vi "FastCMOSTestTrackerModule.vi"() -> ()   [LabVIEW 2011]
uses:
  qtrk/QTrk.llb/QTrkInstance.ctl
  qtrk/QTrk.llb/QTrkLocalizationResult.ctl
  qtrk/QTrk.llb/QTrkLocalizationJob.ctl
  qtrk/QTrk.llb/XYZf.ctl
  mkCameraData.ctl
  CameraConfig.ctl
  Main/Camera/GenericCameraConfigType.ctl
  qtrk/QTrk.llb/QTrkPixelDataType.ctl
  Main/GlobalVariables.vi
  qtrk/QTrk.llb/QTrkDLL.vi
panel:
  in  "Use frame-encoded\ntimestamp":bool
  out "Buffer numbers":i32[](graph)
  out "Buffer Number":i32
  in  "#frames to take":i32=50000
  out "Frame#":u32
  out "Z Result":sgl[](graph)
  out "Unsorted results":T1[](array[typedef])
  out "Results":T1[][](array[typedef])
  out "NumBeads":i32
  out "#frames":u32
  in  "Bead index":i32
  out "XY Result":sgl[][](graph)
  in  "Tracking enabled?":bool
  in  "stop":bool
  out "Status Information : Lost Frames":u32
  out "QTrk Instance":T4
  in  "Run grab sesh":bool
  in  "Stop":bool
  in  "Run":bool
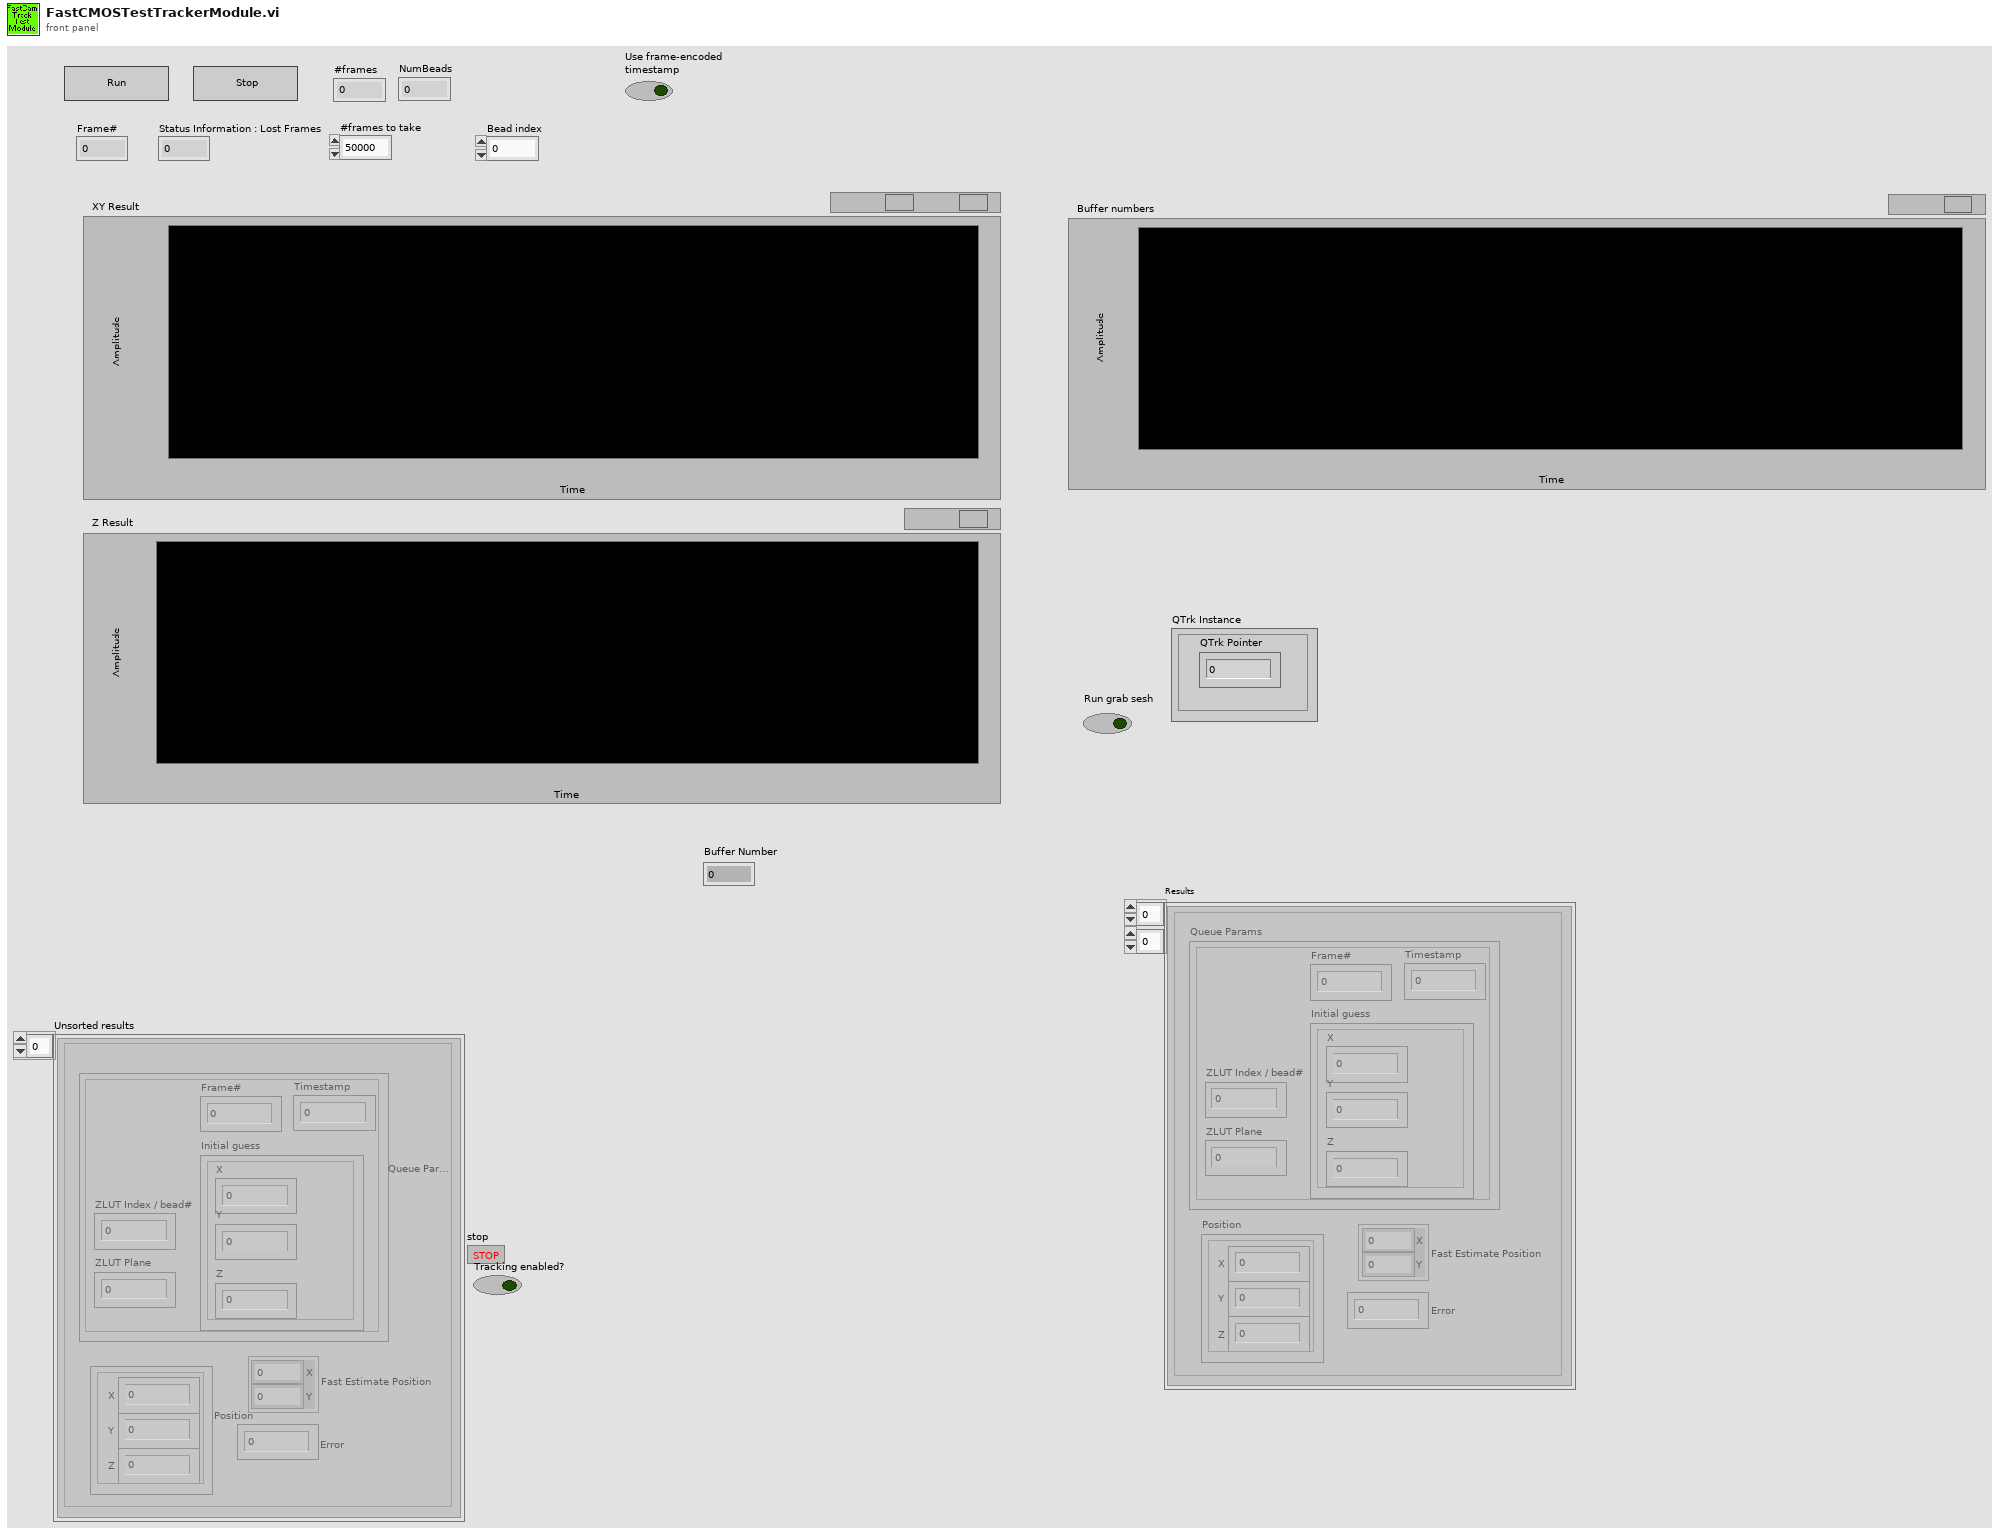
[diagram p1: front panel]
types:
  T1 = typedef "QTrkLocalizationResult.ctl" = cluster{"Queue Params":T2, "Position":T3, "Fast Estimate Position":cluster{"X":sgl, "Y":sgl}, "Error":i32}
  T2 = typedef "QTrkLocalizationJob.ctl" = cluster{"Frame#":u32, "Timestamp":u32, "ZLUT Index / bead#":i32, "ZLUT Plane":i32, "Initial guess":T3}
  T3 = typedef "XYZf.ctl" = cluster{"X":sgl, "Y":sgl, "Z":sgl}
  T4 = typedef "QTrkInstance.ctl" = cluster{"QTrk Pointer":u64}
  T5 = typedef "mkCameraData.ctl" = cluster{"Session":refnum<k11>, "Settings":T6}
  T6 = typedef "CameraConfig.ctl" = cluster{"Gain [1-4]":sgl, "Offset":i16, "Mode":i16, "ROIs":cluster{"X":i32, "Y":i32}[], "ROI Size":cluster{"X":i32, "Y":i32}, "Number of buffers":i32, "Use hardware multiple-ROI?":bool, "GenericCameraConfig":T7}
  T7 = typedef "GenericCameraConfigType.ctl" = cluster{"Framerate (Hz)":i32, "Exposure time (us)":i32, "Image size":cluster{"Width":i32, "Height":i32}, "Number of buffers":i32}
  T8 = enum16{"Use QTrk settings", "Select best device", "Use all devices", "Use custom list"}
  T9 = typedef "CameraInstance.ctl" = cluster{"VI refs":T10, "Camera state":variant}
  T10 = typedef "CameraInterface.ctl" = cluster{"Close":T11, "Get/Set generic config":T12, "Grab":T13, "Show Settings Dialog":T14, "AdjustBeadPos":T15, "Save/load camera settings":T16}
  T11 = typedef "CICloseType.ctl" = refnum<vi>
  T12 = typedef "CIGetSetGenericConfig.ctl" = refnum<vi>
  T13 = typedef "CIGrabType.ctl" = refnum<vi>
  T14 = typedef "CISettingsDlg.ctl" = refnum<vi>
  T15 = typedef "CIAdjustBeadPos.ctl" = refnum<vi>
  T16 = typedef "CISaveLoadSettings.ctl" = refnum<vi>
  T17 = typedef "MeasureConfigType.ctl" = cluster{"Bead locations":cluster{"X":i32, "Y":i32}[], "ROI":i32, "Experiment base path":path, "Image output subdir":string, "Output mode":T18, "Traces output subdir":string, "QTrk Settings":T19, "Tracking Config":T20, "Experiment Name":string, "Program":T23, "ZLUT":sgl[][][], "Camera settings":T7, "Experiment Script":string, "Max frames in memory":i32, "Save traces as binary":bool, "Pixel Calibration Gain Image":string, "Pixel Calibration Offset Image":string, "Use pixel calibration images":bool, "Internal camera settings":string}
  T18 = typedef "MeasureConfigOutputMode.ctl" = enum16{"None", "Track", "SaveImages"}
  T19 = typedef "QTrkSettings.ctl" = cluster{"Image width":i32, "Image height":i32, "Number of threads (CPU based)":i32, "CUDA Device":i32, "COM Background correction factor":sgl, "ZLUT MinRadius":sgl, "ZLUT Radial sample density":sgl, "ZLUT Angular sample density":sgl, "ZLUT ROI Coverage":sgl, "QI Iterations":i32, "QI MinRadius":sgl, "QI Radial sample density":sgl, "QI Angular sample density":sgl, "QI ROI Coverage":sgl, "QI Angular Step \nIteration Factor":sgl, "XCOR Profile Length":i32, "XCOR Profile Width":i32, "XCOR Iterations":i32, "Gaussian 2D Fit Iterations":i32, "Gaussian 2D Sigma (pixels)":sgl}
  T20 = typedef "TrackingConfigType.ctl" = cluster{"Number of steps":i32, "ZLUT stepsize (um)":sgl, "Z correction factor":sgl, "Start piezo Z (um)":sgl, "Pixel size (nm)":sgl, "2D Localization Type":T21, "Z Command (None)":T22, "Z Piezo scale":bool}
  T21 = typedef "QTrkLocalizationType.ctl" = enum16{"Center-of-Mass", "1D Cross-Correlation", "Quadrant Interpolation", "Gaussian 2D MLE", "QI + ZLUTAlign", "ZLUTAlign"}
  T22 = typedef "QTrkZCommandType.ctl" = enum16{"Nothing", "ComputeZ", "BuildRadialZLUT", "BuildImageZLUT", "RadialZLUT+ImageZLUT"}
  T23 = typedef "ExperimentProgramType.ctl" = cluster{"Commands":T24[], "Motor Axis accuracy conditions":T27, "Axis flags":T29}
  T24 = typedef "ExProgCommandType.ctl" = cluster{"cmd":T25, "axis":T26, "value/pos":dbl, "speed":dbl, "name":string}
  T25 = typedef "ExProgCommandEnumType.ctl" = enum16{"wait", "move", "acquire", "idle", "rmove", "when", "section", "stop"}
  T26 = typedef "MotorAxisEnum.ctl" = enum16{"no axis", "magrot", "magpos", "px", "py", "pz", "camx", "camy"}
  T27 = typedef "MotorPosType.ctl" = cluster{"Magnet Z":dbl, "Magnet rotation":dbl, "Camera":T28, "Piezo XY":T28, "Piezo Z":dbl}
  T28 = typedef "XYf.ctl" = cluster{"X":sgl, "Y":sgl}
  T29 = typedef "MotorPosFlagsType.ctl" = cluster{"Magnet Z":bool, "Magnet rotation":bool, "Camera":cluster{"X":bool, "Y":bool}, "Piezo XY":cluster{"X":bool, "Y":bool}, "Piezo Z":bool}
  T30 = enum32{"Map Pixel Pointer", "Unmap Pixel Pointer", "Get Pixels Infos"}
  T31 = typedef "QTrkPixelDataType.ctl" = enum16{"QTrkU8", "QTrkU16", "QTrkFloat"}
  T32 = typedef "QTrkComputedSettings.ctl" = cluster{"QTrk Settings":T19, "Derived settings":cluster{"ZLUT Radial Steps":i32, "ZLUT Angular Steps":i32, "ZLUT Max Radius":sgl, "QI Radial Steps":i32, "QI Angular Steps\nPer Quadrant":i32, "QI Max Radius":sgl}}
  T33 = typedef "IMAQ Image.ctl" = refnum<image>
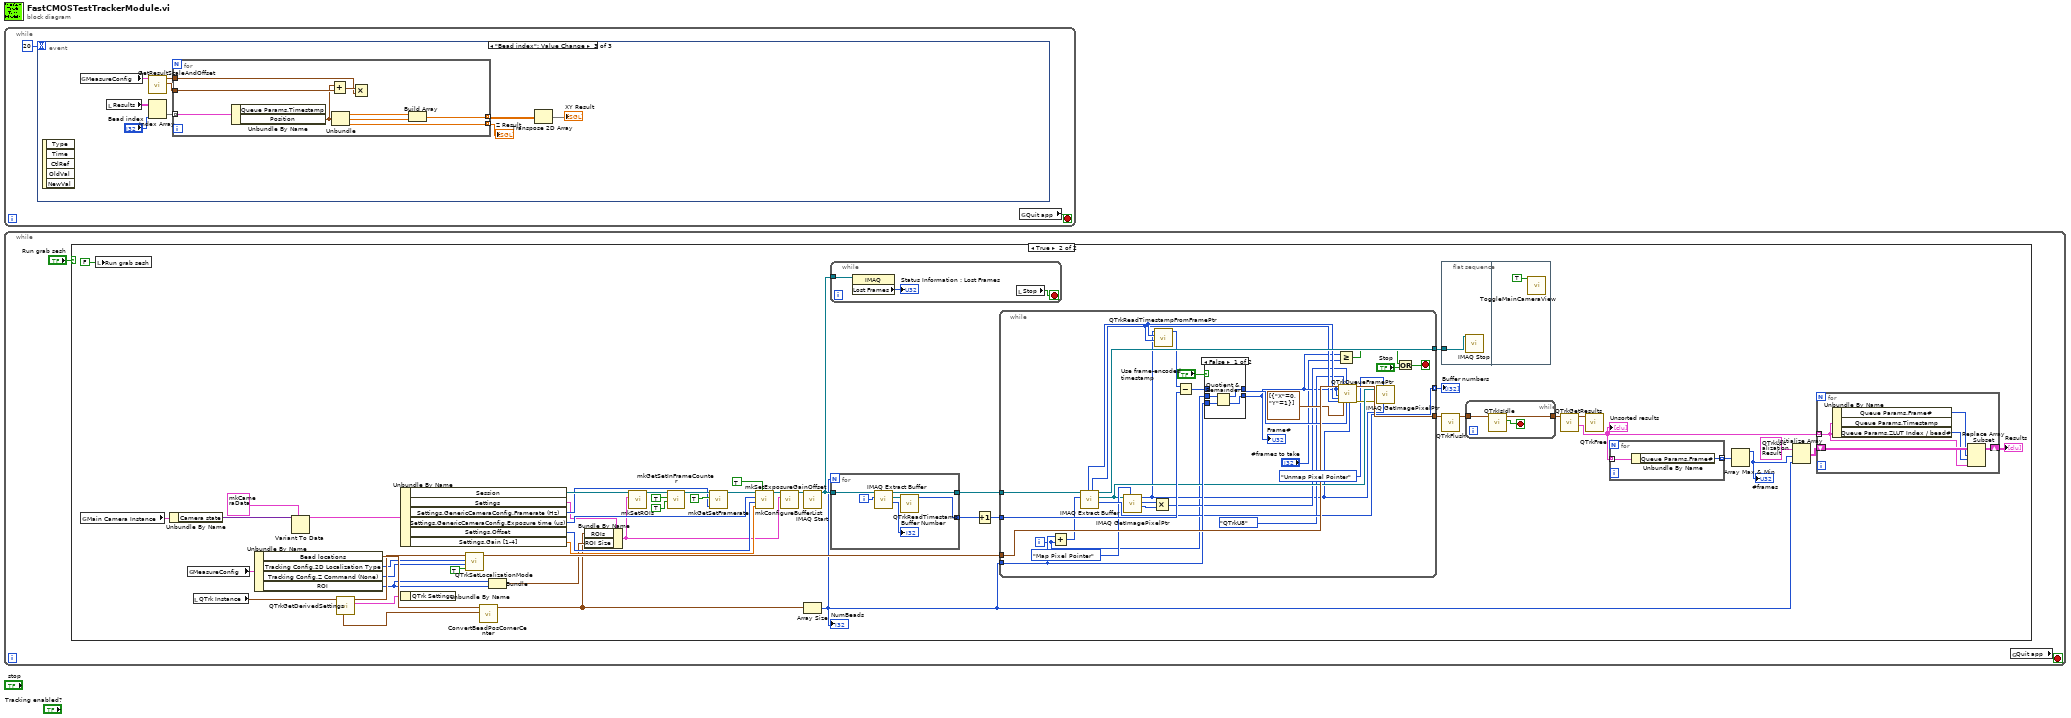
[diagram p0: block diagram]
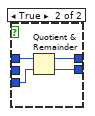
[diagram p3: hidden frame]
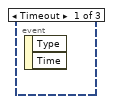
[diagram p4: hidden frame]
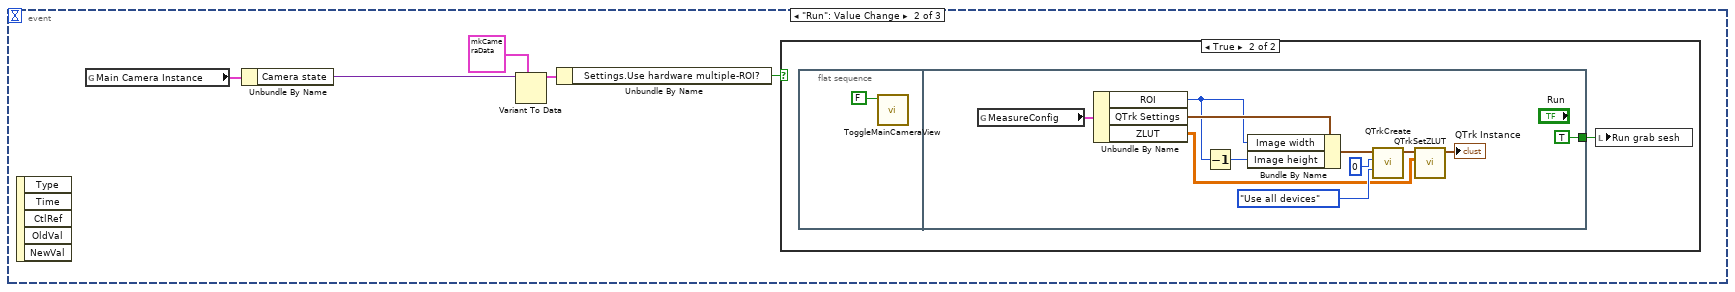
[diagram p5: hidden frame]
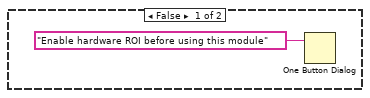
[diagram p6: hidden frame]
diagram:
  n1 = while {
    stop <- w1 stop-if-true
    n2 = event shown="[2] \"Bead index\": Value Change" {
      selector: _ -> [_ _ _]
      dyn-events: _ -> [_ _ _]
      timeout: 20 -> [_ _ _]
      event Timeout {
        n3 = event-data() -> ()  [unwired: 1 in, 2 out]
      }
      event "Run": Value Change {
        n4 = event-data() -> ()  [unwired: 1 in, 5 out]
        n5 = global read "GlobalVariables.vi" "Main Camera Instance"() -> (w5:T9)
        n6 = Unbundle By Name(w5) -> ("Camera state"=w6:variant)
        n7 = Variant To Data(type=T5 {"Session"=refnum, "Settings"={"Gain [1-4]"=1.0, "Offset"=50, "Mode"=6, "ROIs"=[], "ROI Size"={"X"=0, "Y"=0}, "Number of buffers"=40, "Use hardware multiple-ROI?"=FALSE, "GenericCameraConfig"={"Framerate (Hz)"=0, "Exposure time (us)"=0, "Image size"={"Width"=0, "Height"=0}, "Number of buffers"=0}}} ("Camera data"), Variant=w6) -> (data=w4:T5)  [unwired: 1 in, 1 out]
        n8 = Unbundle By Name(w4) -> ("Settings.Use hardware multiple-ROI?"=w3:bool)
        n9 = case shown="True" w3 {
          frame False {
            n10 = One Button Dialog(message="Enable hardware ROI before using this module") -> ()  [unwired: 1 in, 1 out]
          }
          frame True {
            n11 = flat-sequence {
              tunnel: [TRUE ("Run grab sesh")] -> w9
              frame #0 {
                n12 = call "ToggleMainCameraView.vi"("Enable? (T)"=FALSE) -> ()  [unwired: 11 in]
              }
              frame #1 {
                n13 = global read "GlobalVariables.vi" "MeasureConfig"() -> (w21:T17)
                n14 = Unbundle By Name(w21) -> ("ROI"=w16:i32, "QTrk Settings"=w18:T19, "ZLUT"=w11:sgl[][][])
                n15 = Decrement(x=w16) -> (x-1=w17:i32)
                n16 = Bundle By Name(cluster=w18, "Image width"=w16, "Image height"=w17) -> (w15:T19)
                n17 = call "QTrkCreate.vi"("CUDA device selection"=T8."Use all devices", "ROI"=0, "QTrk Settings"=w15) -> ("QTrk Instance"=w13:T4)  [unwired: 2 in, 2 out]
                n18 = call "QTrkSetZLUT.vi"("ZLUT"=w11, "QTrk Instance"=w13) -> ("QTrk Instance"=→"QTrk Instance":T4)  [unwired: 8 in, 1 out]
              }
            }
            n19 = local write "Run grab sesh"(w9) -> ()
          }
        }
      }
      event "Bead index": Value Change {
        n20 = event-data() -> ()  [unwired: 1 in, 5 out]
        n21 = global read "GlobalVariables.vi" "MeasureConfig"() -> (w30:T17)
        n22 = local read "Results"() -> (w29:T1[][])
        n23 = call "GetResultScaleAndOffset.vi"("MeasureConfig"=w30) -> ("offset"=w26:cluster{dbl, dbl, "y":sgl}, "scale"=w25:cluster{sgl, sgl, sgl})  [unwired: 9 in]
        n24 = Index Array(array=w29, index (col)="Bead index") -> (element=w27:T1[])  [unwired: 1 in]
        n25 = for {
          tunnel: w27 -> [w39] mode=indexing
          tunnel: w26 -> [w38]
          tunnel: w25 -> [w36]
          tunnel: [w35] -> w24 mode=indexing
          tunnel: [w32] -> w23 mode=indexing
          n26 = Unbundle By Name(w39) -> ("Position"=w31:T3)  [unwired: 1 out]
          n27 = Add(x=w31, y=w38) -> (x+y=w37:cluster{dbl, dbl, sgl})
          n28 = Unbundle(w31) -> ("X"=w34:sgl, "Y"=w33:sgl, "Z"=w35:sgl)
          n29 = Multiply(x=w37, y=w36) -> ()  [unwired: 1 out]
          n30 = Build Array(w34, w33) -> (w32:sgl[])
        }
        "Z Result" <- w24
        n31 = Transpose 2D Array(2D array=w23) -> (transposed array=→"XY Result":sgl[][])
      }
    }
    n32 = global read "GlobalVariables.vi" "Quit app"() -> (w1:bool)
  }
  n33 = while {
    stop <- w41 stop-if-true
    n34 = case shown="True" "Run grab sesh" {
      frame False {
      }
      frame True {
        n35 = global read "GlobalVariables.vi" "Main Camera Instance"() -> (w92:T9)
        n36 = local write "Run grab sesh"(FALSE ("Run grab sesh")) -> ()
        n37 = Unbundle By Name(w92) -> ("Camera state"=w91:variant)
        n38 = global read "GlobalVariables.vi" "MeasureConfig"() -> (w55:T17)
        n39 = local read "QTrk Instance"() -> (w72:T4)
        n40 = Unbundle By Name(w55) -> ("Bead locations"=w73:cluster{"X":i32, "Y":i32}[], "Tracking Config.2D Localization Type"=w60:T21, "Tracking Config.Z Command (None)"=w61:T22, "ROI"=w45:i32)
        n41 = Variant To Data(type=T5 {"Session"=refnum, "Settings"={"Gain [1-4]"=1.0, "Offset"=50, "Mode"=6, "ROIs"=[], "ROI Size"={"X"=0, "Y"=0}, "Number of buffers"=40, "Use hardware multiple-ROI?"=FALSE, "GenericCameraConfig"={"Framerate (Hz)"=0, "Exposure time (us)"=0, "Image size"={"Width"=0, "Height"=0}, "Number of buffers"=0}}} ("Camera data"), Variant=w91) -> (data=w89:T5)  [unwired: 1 in, 1 out]
        n42 = call "QTrkGetDerivedSettings.vi"("QTrk Instance"=w72) -> ("Derived settings"=w71:T32, "QTrk Instance (out)"=w65:T4, "ROI size"=w70:cluster{"Image width":i32, "Image height":i32})  [unwired: 5 in, 3 out]
        n43 = Unbundle By Name(w89) -> ("Session"=w88:refnum<k11>, "Settings"=w47:T6, "Settings.GenericCameraConfig.Framerate (Hz)"=w81:i32, "Settings.GenericCameraConfig.Exposure time (us)"=w78:i32, "Settings.Offset"=w77:i16, "Settings.Gain [1-4]"=w76:sgl)
        n44 = Unbundle By Name(w71) -> ()  [unwired: 1 out]
        n45 = call "QTrkSetLocalizationMode.vi"("Normalize profile"=TRUE, "Z Command"=w61, "2D Localization Type"=w60, "QTrk Instance"=w65) -> ("QTrk Instance"=w64:T4)  [unwired: 7 in]
        n46 = call "ConvertBeadPosCornerCenter.vi"("ROI Size"=w70, "Center-based bead locations"=w73) -> ("Corner-based bead pos (out)"=w44:cluster{"X":i32, "Y":i32}[])  [unwired: 8 in, 1 out]
        n47 = Bundle("ROI"=w45, "ROI"=w45) -> (w46:cluster{"ROI":i32, "ROI":i32})  [unwired: 1 in]
        n48 = Bundle By Name(cluster=w47, "ROIs"=w44, "ROI Size"=w46) -> (w43:T6)
        n49 = call "mkSetROIs.vi"("Camera in"=w43, "IMAQ Refnum in"=w88) -> ("IMAQ Refnum out"=w86:refnum<k11>)  [unwired: 9 in]
        n50 = call "mkGetSetInFrameCounter.vi"("Set? (F)"=TRUE, "Enable in-frame counter (T)"=TRUE, "IMAQ Refnum in"=w86) -> ("IMAQ Refnum out"=w83:refnum<k11>)  [unwired: 7 in, 1 out]
        n51 = call "mkGetSetFramerate.vi"("Framerate"=w81, "Set? (F)"=TRUE, "IMAQ Refnum out"=w83) -> ("IMAQ Refnum (out)"=w80:refnum<k11>)  [unwired: 5 in, 3 out]
        n52 = call "mkSetExposureGainOffset.vi"("Set? (F)"=TRUE, "Gain [1-4]"=w76, "Offset"=w77, "Exposure time"=w78, "IMAQ Refnum in"=w80) -> ("IMAQ Refnum out"=w75:refnum<k11>)  [unwired: 1 in, 5 out]
        n53 = call "mkConfigureBufferList.vi"("Camera in"=w43, "IMAQ Session"=w75) -> ("IMAQ Session (out)"=w74:refnum<k11>)  [unwired: 9 in]
        n54 = call <vilib>:"IMAQ Start.vi"("IMAQ Session In"=w74) -> ("IMAQ Session Out"=w69:refnum<k11>)  [unwired: 9 in, 1 out]
        n55 = Array Size(array=w44) -> (size(s)=w51:i32)
        "NumBeads" <- w51
        n56 = while {
          tunnel: w69 -> [w107]
          stop <- w105 stop-if-true
          n57 = property class="IMAQ"(reference=w107) -> ("Lost Frames"=→"Status Information : Lost Frames":u32)  [unwired: 1 in, 2 out]
          n58 = local read "Stop"() -> (w105:bool)
        }
        n59 = for {
          N: w51 -> [_]
          tunnel: w69 -> [w112]
          tunnel: [w111] -> w68
          tunnel: [w110] -> w67
          i -> [w109]
          n60 = call <vilib>:"IMAQ Extract Buffer.vi"("Buffer to extract"=w109, "IMAQ Session In"=w112) -> ("Buffer Number"=→"Buffer Number":i32, "Image Out"=w113:T33, "IMAQ Session Out"=w111:refnum<k11>)  [unwired: 4 in, 3 out]
          n61 = call "QTrkReadTimestamp.vi"("Image"=w113) -> ("timestamp"=w110:u32)  [unwired: 10 in]
        }
        n62 = Increment(x=w67) -> (x+1=w66:u32)
        n63 = while {
          tunnel: w68 -> [w143]
          tunnel: w66 -> [w141]
          tunnel: w64 -> [w142]
          tunnel: w51 -> [w135]
          tunnel: [w140] -> w63
          tunnel: [w139] -> w58
          tunnel: [w134] -> w42 mode=indexing
          i -> [w114]
          stop <- w136 stop-if-true
          n64 = Add(x=w135, y=w114) -> (x+y=w116:i32)
          n65 = call <vilib>:"IMAQ Extract Buffer.vi"("Buffer to extract"=w116, "IMAQ Session In"=w143) -> ("Buffer Number"=w134:i32, "Image Out"=w132:T33, "IMAQ Session Out"=w139:refnum<k11>, "Actual Height"=w126:u32, "Actual Width"=w127:u32)  [unwired: 4 in, 1 out]
          n66 = call "IMAQ GetImagePixelPtr"("Function"=T30."Map Pixel Pointer", "Image"=w132) -> ("Pixel Size (Bytes)"=w123:i32, "LineWidth(Pixels)"=w124:i32, "Pixel Pointer out"=w119:u64)  [unwired: 4 in, 3 out]
          n67 = Multiply(x=w124, y=w123) -> (x*y=w122:i32)
          n68 = call "QTrkReadTimestampFromFramePtr.vi"("height"=w126, "width"=w127, "imageptr"=w119) -> ("timestamp"=w131:u32)  [unwired: 8 in]
          n69 = Subtract(x=w131, y=w141) -> (x-y=w130:u32)
          n70 = case shown="False" "Use frame-encoded\ntimestamp" {
            tunnel: w135 -> [w146 w151]
            tunnel: w130 -> [_ w150]
            tunnel: [w145 w149] -> w129
            tunnel: [w144 w148] -> w118
            tunnel: w114 -> [w147 _]
            frame False {
              n71 = Quotient & Remainder(x=w147, y=w146) -> (x-y*floor(x/y)=w145:i32, floor(x/y)=w144:i32)
            }
            frame True {
              n72 = Quotient & Remainder(x=w150, y=w151) -> (x-y*floor(x/y)=w149:u32, floor(x/y)=w148:u32)
            }
          }
          "Frame#" <- w118
          n73 = Greater Or Equal?(x=w118, y="#frames to take") -> (x >= y?=w138:bool)
          n74 = call "QTrkQueueFramePtr.vi"("QTrk Instance"=w142, "frame#"=w118, "timestamp"=w118, "width"=w127, "height"=w126, "Pixel data type"=QTrkPixelDataType."QTrkU8", "ROI Positions (corner-based)"=cluster{"X":i32, "Y":i32}[] [{"X"=0, "Y"=1}], "Image pitch\n(bytes per row)"=w122, "ZLUT Index offset (0)"=w129, "Image Pointer"=w119) -> ("QTrk Instance (out)"=w140:T4, "error out"=w121:errorcluster)  [unwired: 8 in]
          n75 = call "IMAQ GetImagePixelPtr"("Pixel Pointer in"=w119, "Function"=T30."Unmap Pixel Pointer", "error in (no error)"=w121, "Image"=w132) -> ()  [unwired: 2 in, 6 out]
          n76 = Or(x=w138, y="Stop") -> (x .or. y?=w136:bool)
        }
        "Buffer numbers" <- w42
        n77 = flat-sequence {
          tunnel: w58 -> [w100]
          frame #0 {
            n78 = call <vilib>:"IMAQ Stop.vi"("IMAQ Session In"=w100) -> ()  [unwired: 9 in, 2 out]
          }
          frame #1 {
            n79 = call "ToggleMainCameraView.vi"("Enable? (T)"=TRUE) -> ()  [unwired: 11 in]
          }
        }
        n80 = call "QTrkFlush.vi"("QTrk Instance"=w63) -> ("QTrk Instance (out)"=w62:T4)  [unwired: 9 in, 1 out]
        n81 = while {
          tunnel: w62 -> [w104]
          tunnel: [w102] -> w57
          stop <- w103 stop-if-true
          n82 = call "QTrkIsIdle.vi"("QTrk Instance"=w104) -> ("Currently idle?"=w103:bool, "QTrk Instance (out)"=w102:T4)  [unwired: 8 in, 1 out]
        }
        n83 = call "QTrkGetResults.vi"("QTrk Instance"=w57) -> ("results"=w50:T1[], "QTrk Instance"=w56:T4)  [unwired: 4 in, 1 out]
        "Unsorted results" <- w50
        n84 = call "QTrkFree.vi"("QTrk Instance"=w56) -> ()  [unwired: 6 in, 1 out]
        n85 = for {
          tunnel: w50 -> [w99] mode=indexing
          tunnel: [w98] -> w54 mode=indexing
          n86 = Unbundle By Name(w99) -> ("Queue Params.Frame#"=w98:u32)
        }
        n87 = Array Max & Min(array=w54) -> (max value=w52:u32)  [unwired: 3 out]
        "#frames" <- w52
        n88 = Initialize Array(T1 {"Queue Params"={"Frame#"=0, "Timestamp"=0, "ZLUT Index / bead#"=0, "ZLUT Plane"=0, "Initial guess"={"X"=0.0, "Y"=0.0, "Z"=0.0}}, "Position"={"X"=0.0, "Y"=0.0, "Z"=0.0}, "Fast Estimate Position"={"X"=0.0, "Y"=0.0}, "Error"=0} ("Localization Result"), w52, w51) -> (w53:T1[][])
        n89 = for {
          tunnel: w50 -> [w93] mode=indexing
          shift-right: [w96] -> w48
          shift-left: w53 -> [w97]
          n90 = Unbundle By Name(w93) -> ("Queue Params.Frame#"=w95:u32, "Queue Params.ZLUT Index / bead#"=w94:i32)  [unwired: 1 out]
          n91 = Replace Array Subset(array=w97, new element=w93, index (row)=w95, index (col)=w94) -> (w96:T1[][])
        }
        "Results" <- w48
      }
    }
    n92 = global read "GlobalVariables.vi" "Quit app"() -> (w41:bool)
  }
